vi "test_libssh2_sftp_opendir.vi"() -> ()   [LabVIEW 2017, in "integration_tests.lvlib"]
uses:
  integration_tests.lvlib
  libssh2/libssh2_sftp_open_ex.vi
  libssh2/libssh2_sftp_close_handle.vi
  support/support.lvlib
  libssh2/libssh2.lvlib
  <vilib>/PNR/Transparent Assertions/Transparent Assertions/Transparent Assertions.lvlib
panel:
  out "error out":errorcluster
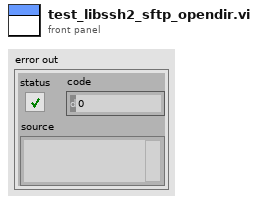
[diagram p1: front panel]
types:
  T1 = typedef "libssh2.lvlib/Session Refnum.ctl" = refnum<k1>
  T2 = typedef "libssh2.lvlib/SFTP Refnum.ctl" = refnum<k1>
  T3 = typedef "libssh2.lvlib/SFTP Handle Refnum.ctl" = refnum<k1>
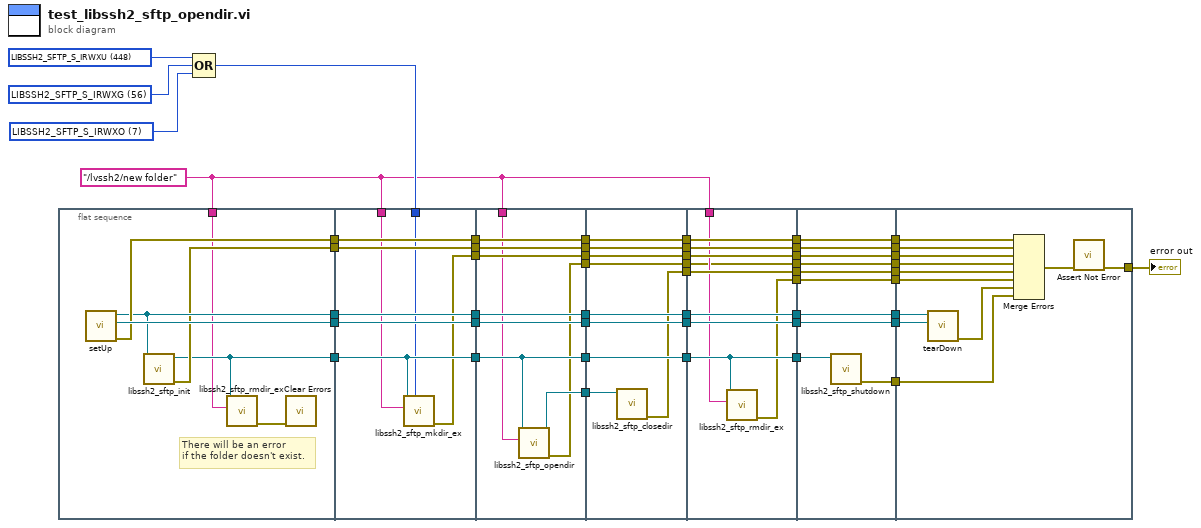
[diagram p0: block diagram]
diagram:
  w7 = "/lvssh2/new folder" ("filename")
  w43 = 7 items=["LIBSSH2_SFTP_S_IRWXU"=448, "LIBSSH2_SFTP_S_IRUSR"=256, "LIBSSH2_SFTP_S_IWUSR"=128, "LIBSSH2_SFTP_S_IXUSR"=64, "LIBSSH2_SFTP_S_IRWXG"=56, "LIBSSH2_SFTP_S_IRGRP"=32, "LIBSSH2_SFTP_S_IWGRP"=16, "LIBSSH2_SFTP_S_IXGRP"=8, "LIBSSH2_SFTP_S_IRWXO"=7, "LIBSSH2_SFTP_S_IROTH"=4, "LIBSSH2_SFTP_S_IWOTH"=2, "LIBSSH2_SFTP_S_IXOTH"=1] ("mode")
  w44 = 56 items=["LIBSSH2_SFTP_S_IRWXU"=448, "LIBSSH2_SFTP_S_IRUSR"=256, "LIBSSH2_SFTP_S_IWUSR"=128, "LIBSSH2_SFTP_S_IXUSR"=64, "LIBSSH2_SFTP_S_IRWXG"=56, "LIBSSH2_SFTP_S_IRGRP"=32, "LIBSSH2_SFTP_S_IWGRP"=16, "LIBSSH2_SFTP_S_IXGRP"=8, "LIBSSH2_SFTP_S_IRWXO"=7, "LIBSSH2_SFTP_S_IROTH"=4, "LIBSSH2_SFTP_S_IWOTH"=2, "LIBSSH2_SFTP_S_IXOTH"=1] ("mode")
  w45 = 448 items=["LIBSSH2_SFTP_S_IRWXU"=448, "LIBSSH2_SFTP_S_IRUSR"=256, "LIBSSH2_SFTP_S_IWUSR"=128, "LIBSSH2_SFTP_S_IXUSR"=64, "LIBSSH2_SFTP_S_IRWXG"=56, "LIBSSH2_SFTP_S_IRGRP"=32, "LIBSSH2_SFTP_S_IWGRP"=16, "LIBSSH2_SFTP_S_IXGRP"=8, "LIBSSH2_SFTP_S_IRWXO"=7, "LIBSSH2_SFTP_S_IROTH"=4, "LIBSSH2_SFTP_S_IWOTH"=2, "LIBSSH2_SFTP_S_IXOTH"=1] ("mode")
  n1 = flat-sequence {
    tunnel: [w56] -> w51
    tunnel: [w58] -> w50
    tunnel: [w57] -> w49
    tunnel: [w55] -> w47
    tunnel: [w54] -> w46
    tunnel: w7 -> [w53]
    tunnel: w51 -> [w66]
    tunnel: w50 -> [w65]
    tunnel: [w66] -> w35
    tunnel: [w65] -> w34
    tunnel: [w62] -> w33
    tunnel: [w64] -> w32
    tunnel: w49 -> [w64]
    tunnel: w47 -> [w63]
    tunnel: [w63] -> w31
    tunnel: w46 -> [w62]
    tunnel: w42 -> [w61]
    tunnel: w7 -> [w60]
    tunnel: [w59] -> w30
    tunnel: w35 -> [w75]
    tunnel: [w75] -> w29
    tunnel: w34 -> [w74]
    tunnel: [w74] -> w28
    tunnel: w33 -> [w70]
    tunnel: [w70] -> w27
    tunnel: w32 -> [w73]
    tunnel: [w73] -> w26
    tunnel: w31 -> [w72]
    tunnel: [w72] -> w25
    tunnel: w30 -> [w71]
    tunnel: [w71] -> w24
    tunnel: w7 -> [w69]
    tunnel: [w68] -> w23
    tunnel: [w67] -> w4
    tunnel: w29 -> [w84]
    tunnel: [w84] -> w21
    tunnel: w28 -> [w83]
    tunnel: [w83] -> w19
    tunnel: w27 -> [w82]
    tunnel: [w82] -> w17
    tunnel: w26 -> [w81]
    tunnel: [w81] -> w15
    tunnel: w25 -> [w80]
    tunnel: [w80] -> w13
    tunnel: w24 -> [w79]
    tunnel: [w79] -> w11
    tunnel: w23 -> [w78]
    tunnel: [w77] -> w9
    tunnel: w4 -> [w76]
    tunnel: [w76] -> w3
    tunnel: w21 -> [w94]
    tunnel: [w94] -> w20
    tunnel: w19 -> [w93]
    tunnel: [w93] -> w18
    tunnel: w17 -> [w88]
    tunnel: [w88] -> w16
    tunnel: w15 -> [w92]
    tunnel: [w92] -> w14
    tunnel: w13 -> [w91]
    tunnel: [w91] -> w12
    tunnel: w11 -> [w90]
    tunnel: [w90] -> w10
    tunnel: w9 -> [w89]
    tunnel: [w89] -> w8
    tunnel: w7 -> [w87]
    tunnel: [w86] -> w6
    tunnel: w3 -> [w85]
    tunnel: [w85] -> w2
    tunnel: w20 -> [w104]
    tunnel: [w104] -> w41
    tunnel: w18 -> [w103]
    tunnel: [w103] -> w40
    tunnel: w16 -> [w100]
    tunnel: w14 -> [w102]
    tunnel: [w102] -> w39
    tunnel: w12 -> [w101]
    tunnel: [w101] -> w38
    tunnel: [w99] -> w37
    tunnel: w10 -> [w98]
    tunnel: [w98] -> w36
    tunnel: w8 -> [w97]
    tunnel: [w97] -> w22
    tunnel: w6 -> [w96]
    tunnel: [w96] -> w5
    tunnel: w2 -> [w95]
    tunnel: [w95] -> w1
    tunnel: w41 -> [w116]
    tunnel: w40 -> [w115]
    tunnel: w39 -> [w114]
    tunnel: [w111] -> w48
    tunnel: w38 -> [w110]
    tunnel: w37 -> [w109]
    tunnel: w36 -> [w108]
    tunnel: w22 -> [w107]
    tunnel: w5 -> [w106]
    tunnel: w1 -> [w105]
    frame #0 {
      # "There will be an error\nif the folder doesn't exist."
      n2 = call "setUp.vi"() -> ("error out"=w57:errorcluster, "connection ID"=w58:refnum<k5>, "session"=w56:T1)  [unwired: 9 in]
      n3 = call "libssh2_sftp_init.vi"("session"=w56) -> ("error out"=w55:errorcluster, "sftp"=w54:T2)  [unwired: 9 in]
      n4 = call "libssh2_sftp_rmdir_ex.vi"("path"=w53, "sftp"=w54) -> ("error out"=w52:errorcluster)  [unwired: 9 in]
      n5 = call <vilib>:"Clear Errors.vi"("error in (no error)"=w52) -> ()  [unwired: 5 in, 2 out]
    }
    frame #1 {
      n6 = call "libssh2_sftp_mkdir_ex.vi"("mode"=w61, "path"=w60, "sftp"=w62) -> ("error out"=w59:errorcluster)  [unwired: 8 in]
    }
    frame #2 {
      n7 = call "libssh2_sftp_opendir.vi"("path"=w69, "sftp"=w70) -> ("error out"=w67:errorcluster, "sftp handle"=w68:T3)  [unwired: 8 in]
    }
    frame #3 {
      n8 = call "libssh2_sftp_closedir.vi"("sftp handle"=w78) -> ("error out"=w77:errorcluster)  [unwired: 10 in]
    }
    frame #4 {
      n9 = call "libssh2_sftp_rmdir_ex.vi"("path"=w87, "sftp"=w88) -> ("error out"=w86:errorcluster)  [unwired: 9 in]
    }
    frame #5 {
      n10 = call "libssh2_sftp_shutdown.vi"("sftp"=w100) -> ("error out"=w99:errorcluster)  [unwired: 10 in]
    }
    frame #6 {
      n11 = call "tearDown.vi"("connection ID"=w115, "session"=w116) -> ("error out"=w113:errorcluster)  [unwired: 9 in]
      n12 = Merge Errors(w114, w110, w108, w105, w107, w106, w113, w109) -> (w112:errorcluster)
      n13 = call <vilib>:"Assert Not Error.vi"("error in (no error)"=w112) -> ("error out"=w111:errorcluster)  [unwired: 10 in]
    }
  }
  n14 = Compound Arithmetic op=OR(w45, w44, w43) -> (w42:i32)
  "error out" <- w48
